vi "Decompress.vi"(8 "Error In":errorcluster, 10 "StringData":string, 11 "reference in":refnum<class "CompressionDecorator.lvclass">) -> (0 "Error Out":errorcluster, 2 "Return(STRING)":string, 3 "reference in":refnum<class "CompressionDecorator.lvclass">)   [LabVIEW 2020, in "CompressionDecorator.lvclass"]
uses:
  CompressionDecorator.lvclass
  <vilib>/zip/NI_Unzip.lvlib
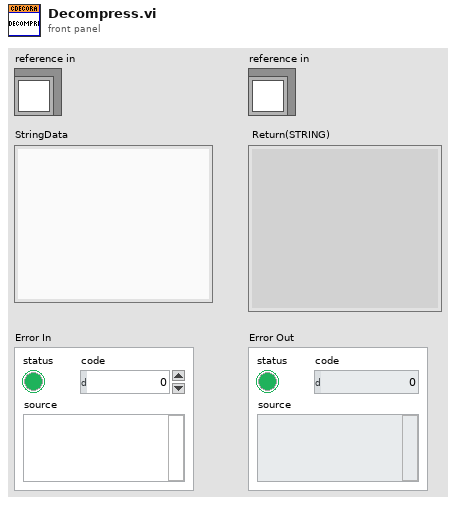
[diagram p1: front panel]
types:
  T1 = typedef "CompressionDecorator.lvclass/ObjectAttributes.ctl" = cluster{"CompLevel":i32}
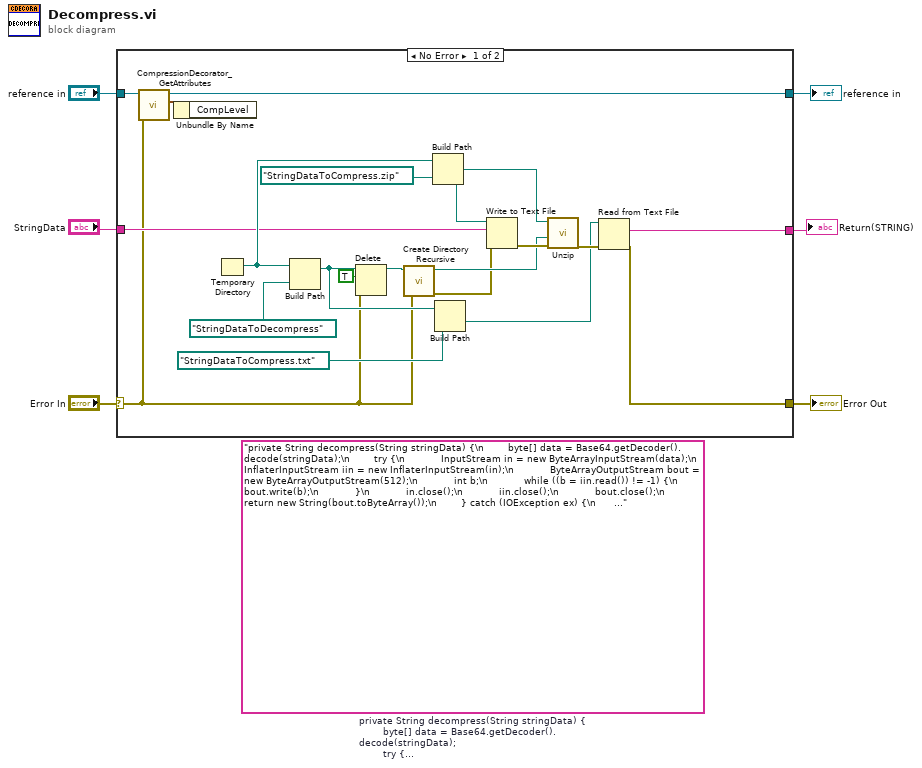
[diagram p0: block diagram]
diagram:
  (unwired) "private String decompress(String stringData) {\n        byte[] data = Base64.getDecoder().decode(stringData);\n        try {\n            InputStream in = new ByteArrayInputStream(data);\n            InflaterInputStream iin = new InflaterInputStream(in);\n            ByteArrayOutputStream bout = new ByteArrayOutputStream(512);\n            int b;\n            while ((b = iin.read()) != -1) {\n                bout.write(b);\n            }\n            in.close();\n            iin.close();\n            bout.close();\n            return new String(bout.toByteArray());\n        } catch (IOException ex) {\n            return null;\n        }\n    }"  # private String decompress(String stringData) {         byte[] data = Base64.getDecoder().decode(stringData);         try {             InputStream in = new ByteArrayInputStream(data);             InflaterInputStream iin = new InflaterInputStream(in);             ByteArrayOutputStream bout = new ByteArrayOutputStream(512);             int b;             while ((b = iin.read()) != -1) {                 bout.write(b);             }             in.close();             iin.close();             bout.close();             return new String(bout.toByteArray());         } catch (IOException ex) {             return null;         }     }
  n1 = case shown="No Error" "Error In" {
    selector: "Error In" -> [w8 w28]
    tunnel: [w9 w28] -> w5
    tunnel: [w25 w27] -> w3
    tunnel: "reference in" -> [w26 w27]
    tunnel: "StringData" -> [w21 _]
    tunnel: [w7 _] -> w1
    frame No Error {
      n2 = call "CompressionDecorator_GetAttributes.vi"("error in (no error)"=w8, "reference in"=w26) -> ("Data"=w24:T1, "reference out"=w25:refnum<class "CompressionDecorator.lvclass">)  [unwired: 6 in, 2 out]
      n3 = Unbundle By Name(w24) -> ()  [unwired: 1 out]
      n4 = Temporary Directory() -> (w23:path)
      n5 = Build Path(base path=w23, name or relative path=path "StringDataToDecompress") -> (appended path=w13:path)
      n6 = Delete(path (use dialog)=w13, entire hierarchy (F)=TRUE, error in=w8) -> (deleted path=w17:path)  [unwired: 2 in, 2 out]
      n7 = call <vilib>:"Create Directory Recursive.vi"("error in (no error)"=w8, "directory"=w17) -> ("error out"=w14:errorcluster, "directory copy"=w15:path)  [unwired: 3 in, 1 out]
      n8 = Build Path(base path=w23, name or relative path=path "StringDataToCompress.zip") -> (appended path=w19:path)
      n9 = Build Path(base path=w13, name or relative path=path "StringDataToCompress.txt") -> (appended path=w10:path)
      n10 = Write to Text File(file (use dialog)=w19, text=w21, error in=w14) -> (error out=w20:errorcluster)  [unwired: 1 in, 2 out]
      n11 = call <vilib>:"Unzip.vi"("error in (no error)"=w20, "Target directory (same as Zip file if empty)"=w15, "Zip file"=w19) -> ("error out"=w11:errorcluster)  [unwired: 6 in, 2 out]
      n12 = Read from Text File(file (use dialog)=w10, error in=w11) -> (text=w7:string, error out=w9:errorcluster)  [unwired: 2 in, 2 out]
    }
    frame Error {
    }
  }
  "Error Out" <- w5
  "reference in" <- w3
  "Return(STRING)" <- w1
